vi "chm test.vi"() -> ()   [LabVIEW 2014]
uses:
  <vilib>/Utility/sysdir.llb/System Directory Type.ctl
  Config Global.vi
  Configuration Tool.lvlib
panel:
  out "resulting string":string
  in  "WebBrowser":refnum<k7>(container)
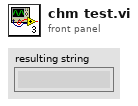
[diagram p1: front panel]
types:
  T1 = typedef "System Directory Type.ctl" = i32
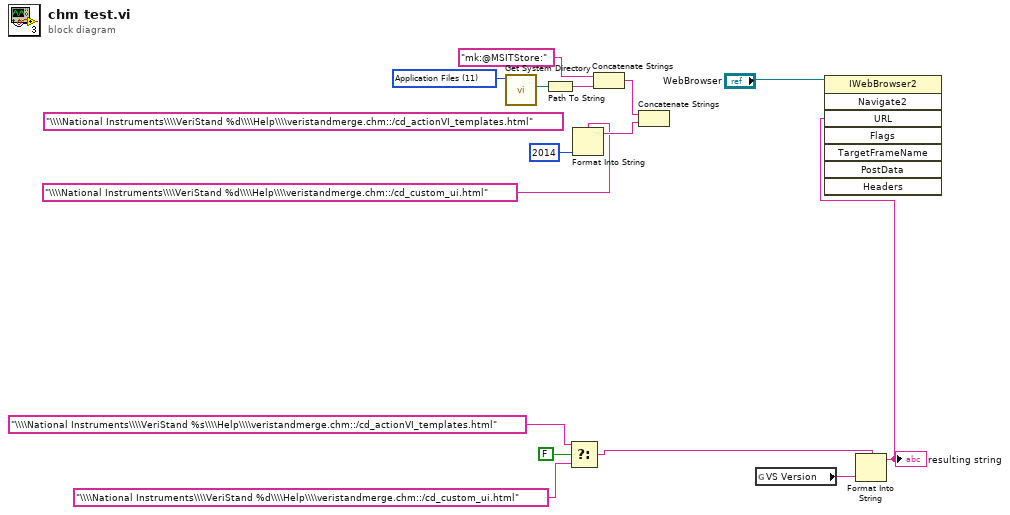
[diagram p0: block diagram]
diagram:
  (unwired) "\\\\National Instruments\\\\VeriStand %d\\\\Help\\\\veristandmerge.chm::/cd_actionVI_templates.html"
  w15 = T1 11 items=["User Home"=0, "User Desktop"=1, "User Documents"=2, "User Application Data"=3, "User Preferences"=4, "User Temporary"=5, "Public Documents"=6, "Public Application Data"=7, "Public Preferences"=8, "Public Cache"=13, "System Core Libraries"=9, "System Installed Libraries"=10, "Application Files"=11, "Boot Volume Root"=12] ("system directory type")
  n1 = call <vilib>:"Get System Directory.vi"("system directory type"=w15) -> ("system directory"=w13:path)  [unwired: 10 in]
  n2 = Path To String(path=w13) -> (string=w12:string)
  n3 = Select(t="\\\\National Instruments\\\\VeriStand %s\\\\Help\\\\veristandmerge.chm::/cd_actionVI_templates.html", s=FALSE, f="\\\\National Instruments\\\\VeriStand %d\\\\Help\\\\veristandmerge.chm::/cd_custom_ui.html") -> (s? t:f=w6:string)
  n4 = Format Into String(format string="\\\\National Instruments\\\\VeriStand %d\\\\Help\\\\veristandmerge.chm::/cd_custom_ui.html", 2014) -> (resulting string=w9:string)  [unwired: 2 in, 1 out]
  n5 = Concatenate Strings("mk:@MSITStore:" ("concatenated string"), w12) -> (w10:string)
  n6 = Concatenate Strings(w10, w9) -> ()  [unwired: 1 out]
  n7 = global read "Config Global.vi" "VS Version"() -> (w4:string)
  n8 = Format Into String(format string=w6, w4) -> (resulting string=w1:string)  [unwired: 2 in, 1 out]
  "resulting string" <- w1
  n9 = invoke class="IWebBrowser2" method="Navigate2"(reference="WebBrowser", "URL"=w1) -> ()  [unwired: 6 in, 8 out]
